vi "http tls handle content data.vi"(7 "buffer in":string, 9 "server properties":T4={"max url size"=8000, "max header"=8000, "timeout ms"=5000, "max data size"=104857600}, 10 "application request":T1, 11 "lvlibretls connection in":refnum<class "lvlibretls connection.lvclass">) -> (0 "connection error":bool, 2 "application request out":T1, 5 "buffer out":string)   [LabVIEW 2016, in "Basic HTTPS server.lvclass"]
uses:
  Basic HTTPS server.lvclass
  http request.ctl
  http method.ctl
  HTTP headers/http header data.ctl
  http server properties.ctl
  lvlibtls/socket connection/lvlibretls connection.lvclass
  http chunked encoding state.ctl
  <vilib>/dlg_ctls.llb/Space Constant.vi
  HTTP headers/http add header to set.vi
  HTTP headers/http headers.lvlib
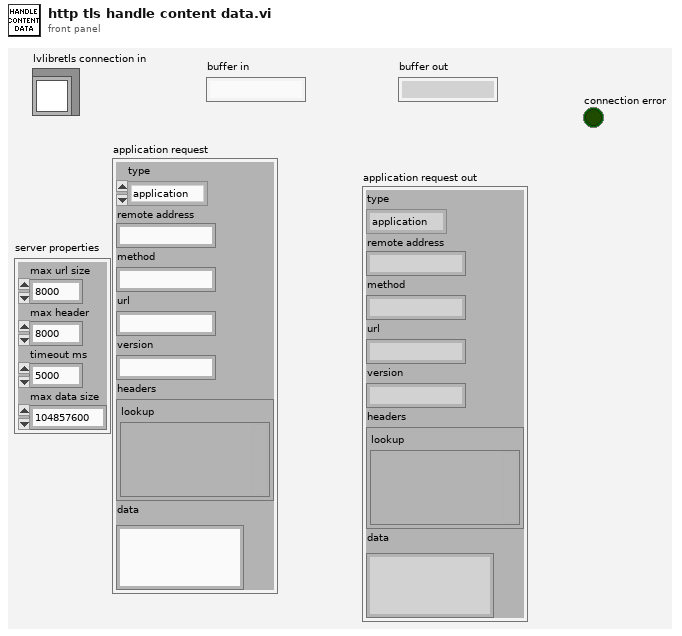
[diagram p1: front panel]
types:
  T1 = typedef "Basic HTTPS server.lvclass/http request.ctl" = cluster{"type":T2, "remote address":string, "method":string, "url":string, "version":string, "headers":T3, "data":string}
  T2 = typedef "Basic HTTPS server.lvclass/http method.ctl" = enum16{"application", "error", "upgrade"}
  T3 = typedef "http headers.lvlib/http header data.ctl" = cluster{"lookup":variant}
  T4 = typedef "Basic HTTPS server.lvclass/http server properties.ctl" = cluster{"max url size":i32, "max header":i32, "timeout ms":i32, "max data size":i32}
  T5 = typedef "Basic HTTPS server.lvclass/http chunked encoding state.ctl" = enum16{"length", "data", "trailer"}
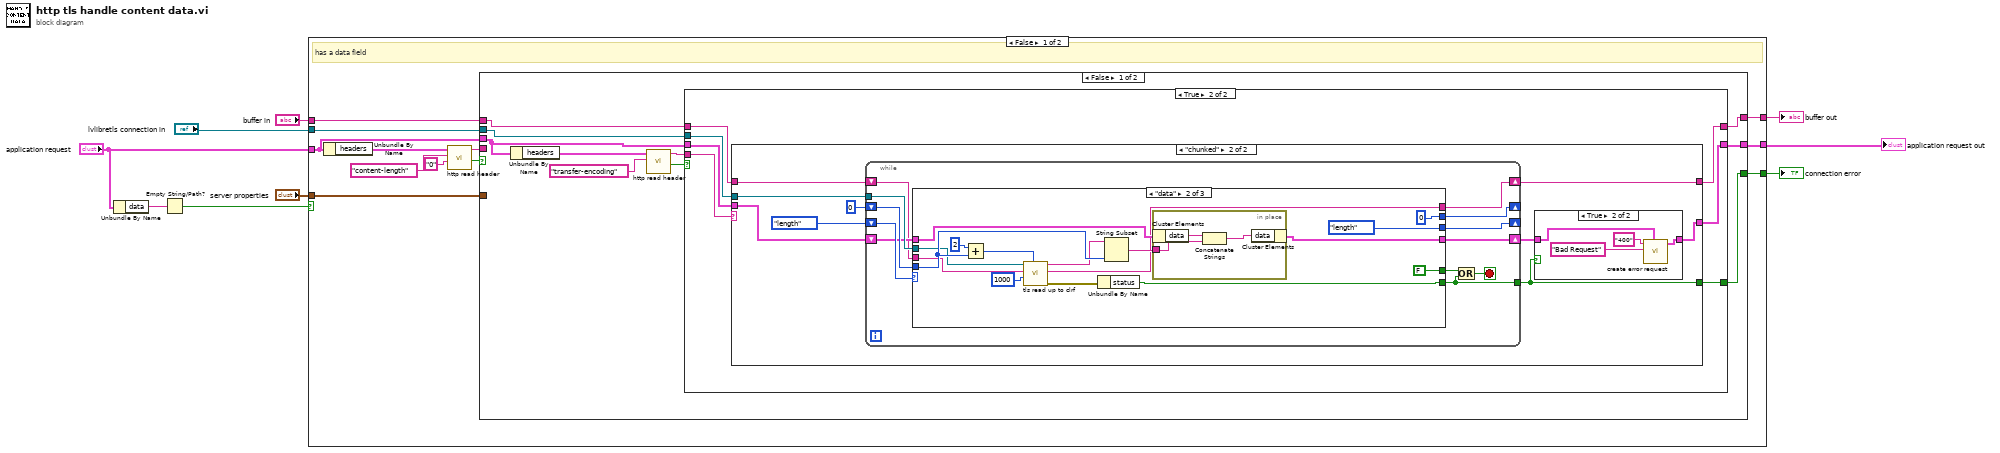
[diagram p0: block diagram]
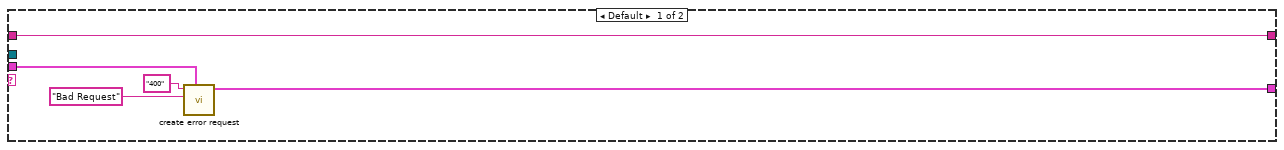
[diagram p3: hidden frame]
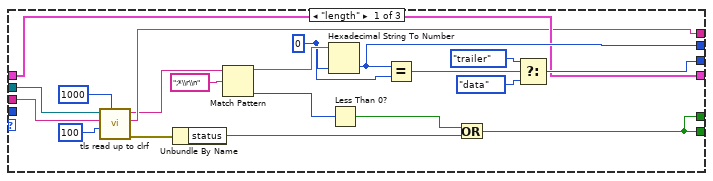
[diagram p5: hidden frame]
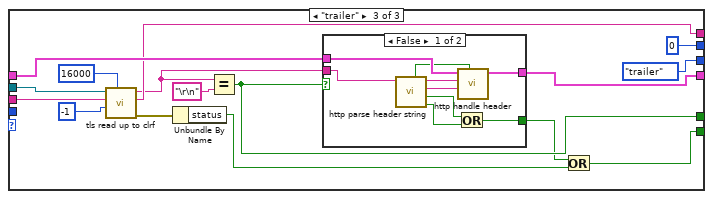
[diagram p6: hidden frame]
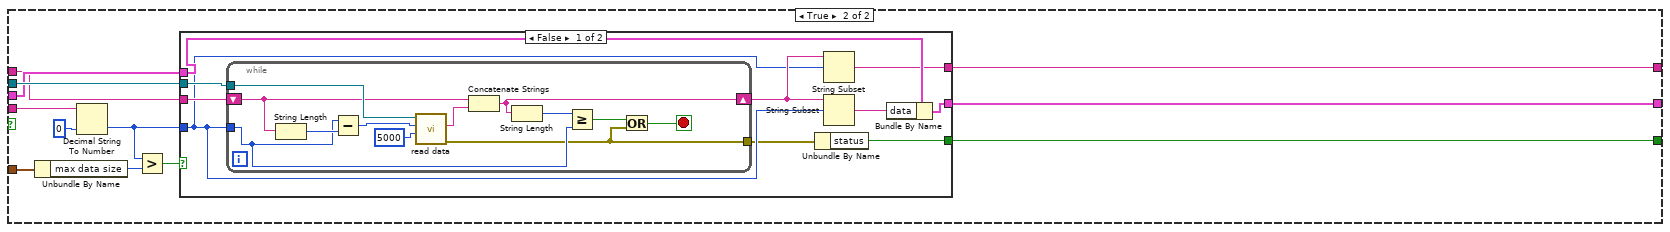
[diagram p8: hidden frame]
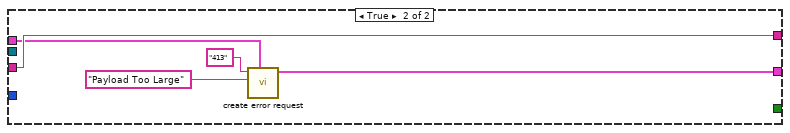
[diagram p9: hidden frame]
diagram:
  n1 = Unbundle By Name("application request") -> ("data"=w7:string)
  n2 = Empty String/Path?(string/path=w7) -> (empty?=w6:bool)
  n3 = case shown="False" w6 {
    tunnel: "lvlibretls connection in" -> [w21 _]
    tunnel: "server properties" -> [w20 _]
    tunnel: "application request" -> [w19 w176]
    tunnel: [w12 w177] -> w4
    tunnel: "buffer in" -> [w13 w177]
    tunnel: [w11 w176] -> w2
    tunnel: [w10 _] -> w1
    frame False {
      # "has a data field"
      n4 = Unbundle By Name(w19) -> ("headers"=w18:T3)
      n5 = call "http read header.vi"("default value"="0", "header field name"="content-length" ("name"), "headers"=w18) -> ("found"=w16:bool, "value"=w15:string)  [unwired: 7 in]
      n6 = case shown="False" w16 {
        tunnel: w19 -> [w31 w142]
        tunnel: w21 -> [w30 w147]
        tunnel: w20 -> [_ w146]
        tunnel: w15 -> [_ w141]
        tunnel: w13 -> [w25 w140]
        tunnel: [w24 w139] -> w12
        tunnel: [w23 w138] -> w11
        tunnel: [w22 w137] -> w10
        frame False {
          n7 = Unbundle By Name(w31) -> ("headers"=w29:T3)
          n8 = call "http read header.vi"("header field name"="transfer-encoding" ("name"), "headers"=w29) -> ("found"=w27:bool, "value"=w26:string)  [unwired: 8 in]
          n9 = case shown="True" w27 {
            tunnel: w31 -> [w32 w39]
            tunnel: w30 -> [_ w40]
            tunnel: w26 -> [_ w38]
            tunnel: w25 -> [w33 w37]
            tunnel: [w33 w36] -> w24
            tunnel: [w32 w35] -> w23
            tunnel: [_ w34] -> w22
            frame False {
              # "apparently no data"
            }
            frame True {
              n10 = case shown="\"chunked\"" w38 {
                tunnel: w39 -> [w43 w51]
                tunnel: w40 -> [_ w53]
                tunnel: w37 -> [w42 w49]
                tunnel: [w42 w48] -> w36
                tunnel: [w41 w47] -> w35
                tunnel: [_ w46] -> w34
                frame Default {
                  n11 = call "create error request.vi"("incoming request"=w43, "reason"="Bad Request" ("status string"), "code"="400") -> ("element"=w41:T1)  [unwired: 8 in]
                }
                frame "chunked" {
                  n12 = while {
                    shift-right: [w69] -> _
                    shift-left: http_chunked_encoding_state."length" -> [w71]
                    tunnel: w53 -> [w70]
                    shift-right: [w67] -> _
                    shift-left: 0 ("default (0 I32)") -> [w66]
                    shift-right: [w64] -> w50
                    shift-left: w51 -> [w65]
                    tunnel: [w62] -> w46
                    shift-right: [w60] -> w48
                    shift-left: w49 -> [w61]
                    stop <- w63 stop-if-true
                    n13 = case shown="\"data\"" w71 {
                      tunnel: w70 -> [w73 w98 w117]
                      tunnel: [w83 http_chunked_encoding_state."length" http_chunked_encoding_state."trailer"] -> w69
                      tunnel: [w80 FALSE w122] -> w68
                      tunnel: [w88 0 0] -> w67
                      tunnel: w66 -> [_ w106 _]
                      tunnel: w65 -> [w82 w100 w120]
                      tunnel: [w82 w99 w121] -> w64
                      tunnel: [w80 w101 w119] -> w62
                      tunnel: w61 -> [w78 w97 w116]
                      tunnel: [w77 w96 w115] -> w60
                      frame "length" {
                        w89 = 0 ("default (0 I32)")
                        n14 = call "tls read up to clrf.vi"("max size"=1000 ("bytes to read"), "timeout ms"=100 ("timeout ms (25000)"), "buffer in"=w78, "lvlibretls connection in"=w73) -> ("error out"=w75:errorcluster, "buffer out"=w77:string, "line out"=w76:string)  [unwired: 5 in]
                        n15 = Unbundle By Name(w75) -> ("status"=w79:bool)
                        n16 = Match Pattern(string=w76, regular expression=";*\\r\\n") -> (before substring=w90:string, offset past match=w87:i32)  [unwired: 1 in, 2 out]
                        n17 = Hexadecimal String To Number(string=w90, default (0uL)=w89) -> (number=w88:i32)  [unwired: 1 in, 1 out]
                        n18 = Less Than 0?(x=w87) -> (x < 0?=w81:bool)
                        n19 = Equal?(x=w88, y=w89) -> (x = y?=w86:bool)
                        n20 = Or(x=w81, y=w79) -> (x .or. y?=w80:bool)
                        n21 = Select(t=http_chunked_encoding_state."trailer", s=w86, f=http_chunked_encoding_state."data") -> (s? t:f=w83:T5)
                      }
                      frame "data" {
                        n22 = Add(x=2, y=w106) -> (x+y=w94:i32)
                        n23 = call "tls read up to clrf.vi"("max size"=w94, "timeout ms"=1000 ("timeout ms (25000)"), "buffer in"=w97, "lvlibretls connection in"=w98) -> ("error out"=w92:errorcluster, "buffer out"=w96:string, "line out"=w93:string)  [unwired: 5 in]
                        n24 = Unbundle By Name(w92) -> ("status"=w101:bool)
                        n25 = String Subset(string=w93, length (rest)=w106) -> (substring=w105:string)  [unwired: 1 in]
                        n26 = in-place {
                          in-place-border: w105 -> [w110]
                          n27 = in-place-cluster #1(w100) -> ("data"=w109:string)
                          n28 = Concatenate Strings(w109, w110) -> (w108:string)
                          n29 = in-place-cluster #1("data"=w108) -> (w99:T1)
                        }
                      }
                      frame "trailer" {
                        n30 = call "tls read up to clrf.vi"("max size"=16000 ("bytes to read"), "timeout ms"=-1 ("timeout ms (25000)"), "buffer in"=w116, "lvlibretls connection in"=w117) -> ("error out"=w113:errorcluster, "buffer out"=w115:string, "line out"=w114:string)  [unwired: 5 in]
                        n31 = Unbundle By Name(w113) -> ("status"=w125:bool)
                        n32 = Equal?(x=w114, y="\r\n" ("x")) -> (x = y?=w122:bool)
                        n33 = case shown="False" w122 {
                          tunnel: [w135 w136] -> w121
                          tunnel: w120 -> [w134 w136]
                          tunnel: [w130 _] -> w118
                          tunnel: w114 -> [w131 _]
                          frame False {
                            n34 = call "http parse header string.vi"("raw string"=w131) -> ("no field name"=w129:bool, "no crlf"=w133:bool, "header field data"=w132:string, "header field name"=w128:string, "continuation"=w127:bool)  [unwired: 6 in]
                            n35 = Or(x=w133, y=w129) -> (x .or. y?=w130:bool)
                            n36 = call "http handle header.vi"("continuation"=w127, "header field data"=w132, "header field name"=w128, "application request in"=w134) -> ("application request out"=w135:T1)  [unwired: 7 in]
                          }
                          frame True {
                          }
                        }
                        n37 = Or(x=w118, y=w125) -> (x .or. y?=w119:bool)
                      }
                    }
                    n38 = Or(x=w68, y=w62) -> (x .or. y?=w63:bool)
                  }
                  n39 = case shown="True" w46 {
                    tunnel: w50 -> [w55 w57]
                    tunnel: [w55 w56] -> w47
                    frame False {
                    }
                    frame True {
                      n40 = call "create error request.vi"("incoming request"=w57, "reason"="Bad Request" ("status string"), "code"="400") -> ("element"=w56:T1)  [unwired: 8 in]
                    }
                  }
                }
              }
            }
          }
        }
        frame True {
          n41 = Unbundle By Name(w146) -> ("max data size"=w145:i32)
          n42 = Decimal String To Number(string=w141, default (0L)=0 ("default (0 I32)")) -> (number=w144:i32)  [unwired: 1 in, 1 out]
          n43 = Greater?(x=w144, y=w145) -> (0:w143:bool)
          n44 = case shown="False" w143 {
            tunnel: w147 -> [w157 _]
            tunnel: w142 -> [w158 w171]
            tunnel: w144 -> [w154 _]
            tunnel: w140 -> [w156 w173]
            tunnel: [w153 w173] -> w139
            tunnel: [w151 w172] -> w138
            tunnel: [w149 _] -> w137
            frame False {
              n45 = while {
                tunnel: w157 -> [w170]
                shift-right: [w162] -> w155
                shift-left: w156 -> [w167]
                tunnel: w154 -> [w165]
                tunnel: [w159] -> w150
                stop <- w161 stop-if-true
                n46 = String Length(string=w167) -> (length=w166:i32)
                n47 = Subtract(x=w165, y=w166) -> (x-y=w168:i32)
                n48 = call "read data.vi"("timeout"=5000, "max size"=w168, "lvlibretls connection in"=w170) -> ("error out"=w159:errorcluster, "data"=w164:string)  [unwired: 6 in, 1 out]
                n49 = Concatenate Strings(w167, w164) -> (w162:string)
                n50 = String Length(string=w162) -> (length=w163:i32)
                n51 = Greater Or Equal?(x=w163, y=w165) -> (x >= y?=w160:bool)
                n52 = Or(x=w160, y=w159) -> (x .or. y?=w161:bool)
              }
              n53 = Unbundle By Name(w150) -> ("status"=w149:bool)
              n54 = String Subset(string=w155, offset (0)=w154) -> (substring=w153:string)  [unwired: 1 in]
              n55 = String Subset(string=w155, offset (0)=w154) -> (substring=w152:string)  [unwired: 1 in]
              n56 = Bundle By Name(cluster=w158, "data"=w152) -> (w151:T1)
            }
            frame True {
              n57 = call "create error request.vi"("incoming request"=w171, "reason"="Payload Too Large" ("status string"), "code"="413") -> ("element"=w172:T1)  [unwired: 8 in]
            }
          }
        }
      }
    }
    frame True {
      # "no data"
    }
  }
  "buffer out" <- w4
  "application request out" <- w2
  "connection error" <- w1
